vi "msize.vi"(8 "error in (no error)":errorcluster, 11 "para0":u32) -> (0 "error out":errorcluster, 2 "function return":u64, 3 "para0 out":u32)   [LabVIEW 2020, in "sqlite3.lvlib"]
uses:
  sqlite3.lvlib
  errstr.vi
  bin/sqlite3_64.dll
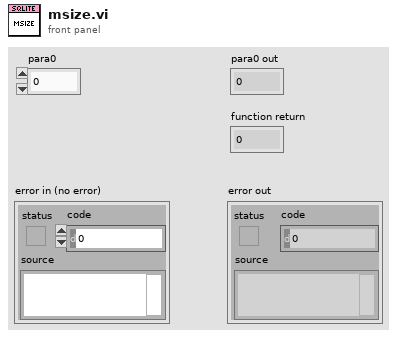
[diagram p1: front panel]
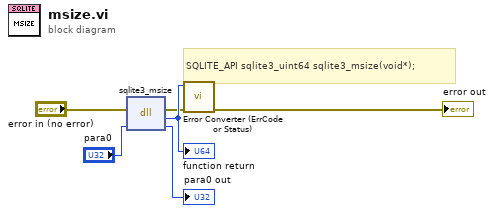
[diagram p0: block diagram]
diagram:
  # "SQLITE_API sqlite3_uint64 sqlite3_msize(void*);"
  n1 = dll-call lib="D:/Project/Labview-Projects/database-configuration/externals/sqlite3/Source/bin/sqlite3_*.*" fn="sqlite3_msize"(error in="error in (no error)", "para0"="para0") -> (error out=w2:errorcluster, w6:u64, "para0"=→"para0 out":u32)  [unwired: 2 in, 1 out]
  "function return" <- w6
  n2 = call "Error Converter (ErrCode or Status).vi"("error in (no error)"=w2, "error code"=w6) -> ("error out"=→"error out":errorcluster)  [unwired: 9 in]
